vi "VI Package to SBOM Component.vi"(6 "Additional License Aliases (empty = defaults only)":T1[](array[typedef]), 8 "error in (no error)":errorcluster, 11 "VIP Information":T2) -> (0 "error out":errorcluster, 3 "CycloneDX Component":refnum<class "CycloneDX Component.lvclass">)   [LabVIEW 2017, in "VIP SBOM Support.lvlib"]
doc: "Converts VI package information into a CycloneDX SBOM component."
uses:
  VIP SBOM Support.lvlib
  <vilib>/JKI/VIPM API/command-line/support/Library Contents Cluster_vipm_api.ctl
  CycloneDX/CycloneDX Component/CycloneDX Component.lvclass
  C:/LabVIEW Working Directory/labview-cyclonedx-sbom/Source/CycloneDX/CycloneDX JSON/CycloneDX JSON.lvclass
  VIP License Alias.ctl
  CycloneDX/CycloneDX JSON/CycloneDX Types.ctl
  CycloneDX/CycloneDX JSON/CycloneDX JSON.lvclass
  <vilib>/JKI/VIPM API/VIPM API_vipm_api.lvlib
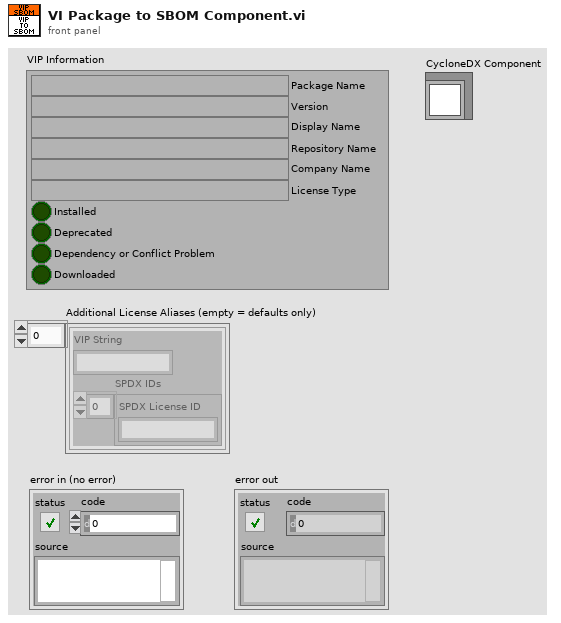
[diagram p1: front panel]
types:
  T1 = typedef "VIP SBOM Support.lvlib/VIP License Alias.ctl" = cluster{"VIP String":string, "SPDX IDs":string[]}
  T2 = typedef "VIPM API_vipm_api.lvlib/Library Contents Cluster_vipm_api.ctl" = cluster{"Package Name":string, "Version":string, "Display Name":string, "Repository Name":string, "Company Name":string, "License Type":string, "Installed":bool, "Deprecated":bool, "Dependency or Conflict Problem":bool, "Downloaded":bool}
  T3 = typedef "LabVIEW CycloneDX SBOM.lvlib/CycloneDX JSON.lvclass/CycloneDX Types.ctl" = enum16{"application", "framework", "library", "container", "platform", "operating-system", "device", "device-driver", "firmware", "file", "machine-learning-model", "data"}
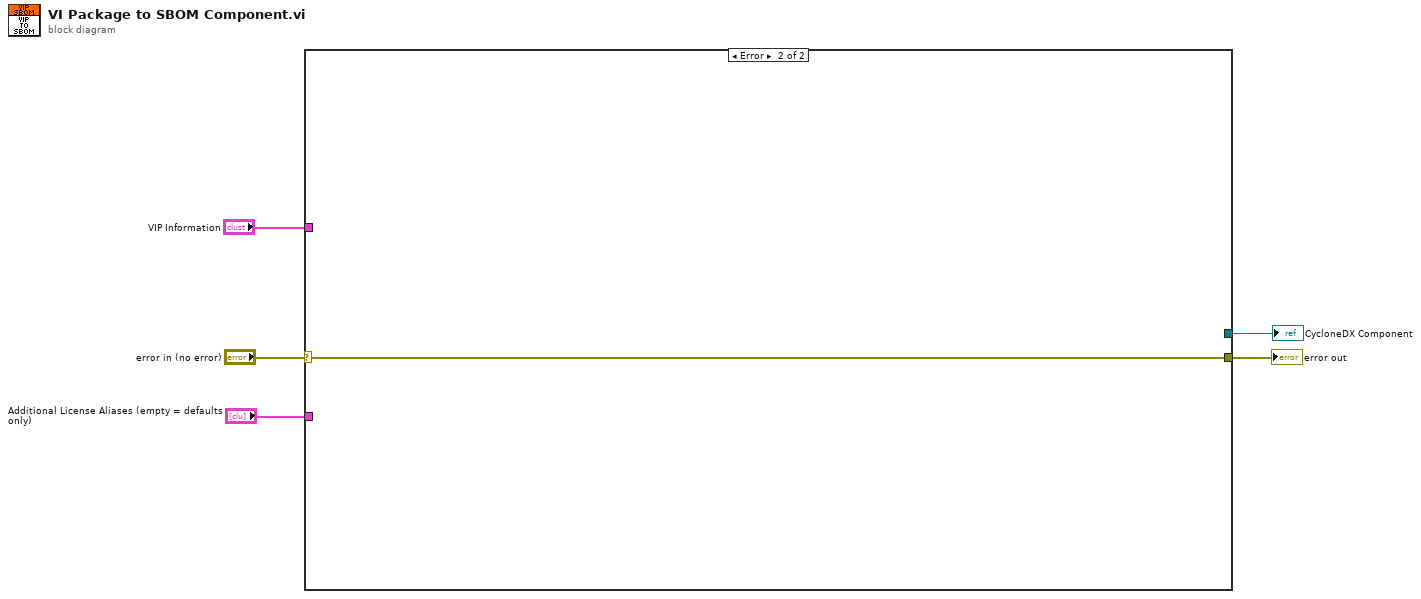
[diagram p0: block diagram]
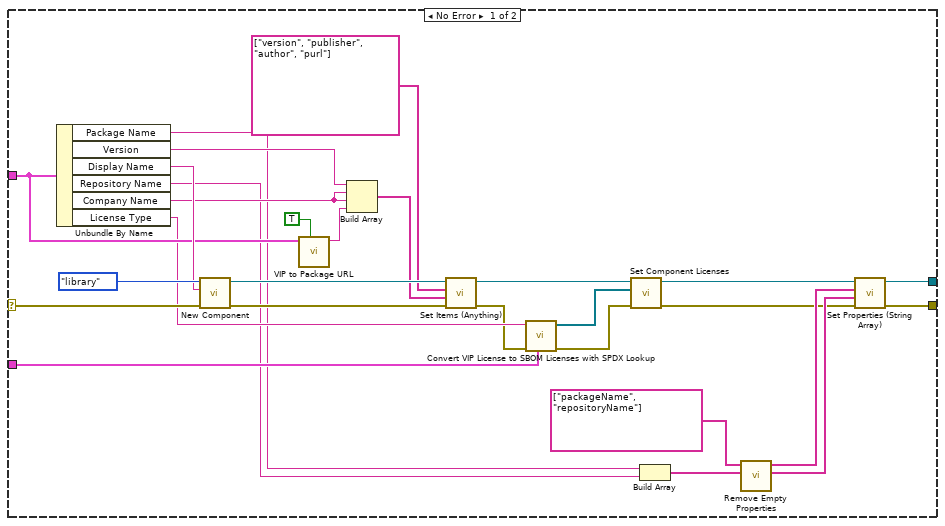
[diagram p2: hidden frame]
diagram:
  n1 = case shown="Error" "error in (no error)" {
    selector: "error in (no error)" -> [w33 w34]
    tunnel: "VIP Information" -> [w24 _]
    tunnel: "Additional License Aliases (empty = defaults only)" -> [w16 _]
    tunnel: [w12 _] -> w2
    tunnel: [w10 w34] -> w1
    frame No Error {
      n2 = Unbundle By Name(w24) -> ("Package Name"=w8:string, "Version"=w27:string, "Display Name"=w31:string, "Repository Name"=w7:string, "Company Name"=w26:string, "License Type"=w20:string)
      n3 = call "New Component.vi"("error in (no error)"=w33, "name"=w31, "type"=CycloneDX_Types."library") -> ("error out"=w30:errorcluster, "CycloneDX Component out"=w29:refnum<class "CycloneDX Component.lvclass">)  [unwired: 7 in]
      n4 = call "VIP to Package URL.vi"("Include Repository?"=TRUE ("Include Repositories?"), "VIP Information"=w24) -> ("VIP Package URL"=w23:string)  [unwired: 9 in]
      n5 = Build Array(w27, w26, w26, w23) -> (w25:string[])
      n6 = call "Set Items (Anything).vi"("error in (no error)"=w30, "Value"=w25, "Item Paths"=string[] ["version", "publisher", "author", "purl"], "CycloneDX SBOM in"=w29) -> ("error out"=w18:errorcluster, "CycloneDX SBOM out"=w21:refnum<class "CycloneDX Component.lvclass">)  [unwired: 6 in]
      n7 = call "Convert VIP License to SBOM Licenses with SPDX Lookup.vi"("Additional Custom Aliases (empty = defaults only)"=w16, "error in (no error)"=w18, "VIP License Type in"=w20) -> ("error out"=w17:errorcluster, "License(s) out"=w19:refnum<class "CycloneDX License.lvclass">[])  [unwired: 7 in]
      n8 = call "Set Component Licenses.vi"("error in (no error)"=w17, "License(s)"=w19, "CycloneDX Component in"=w21) -> ("error out"=w11:errorcluster, "CycloneDX Component out"=w13:refnum<class "CycloneDX Component.lvclass">)  [unwired: 7 in]
      n9 = Build Array(w8, w7) -> (w6:string[])
      n10 = call "Remove Empty Properties.vi"("Values in"=w6, "Names in"=string[] ["packageName", "repositoryName"]) -> ("Values out"=w14:string[], "Names out"=w15:string[])  [unwired: 8 in]
      n11 = call "Set Properties (String Array).vi"("error in (no error)"=w11, "values (string)"=w14, "names"=w15, "CycloneDX JSON in"=w13) -> ("error out"=w10:errorcluster, "CycloneDX JSON out"=w12:refnum<class "CycloneDX Component.lvclass">)  [unwired: 6 in]
    }
    frame Error {
    }
  }
  "CycloneDX Component" <- w2
  "error out" <- w1
